vi "RT - Initialize Control Mode.vi"(8 "error in":errorcluster) -> (0 "error out":errorcluster)   [LabVIEW 2014]
uses:
  Controls/DLT State.ctl
  Controls/IT State.ctl
  Controls/OT State.ctl
  Controls/TWT State.ctl
  Controls/Clean State.ctl
  Controls/DL State.ctl
  Controls/Clamp State.ctl
  Controls/BR State.ctl
  Controls/ConfigCalibration.ctl
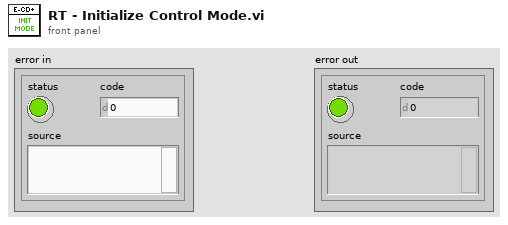
[diagram p1: front panel]
types:
  T1 = typedef "ConfigCalibration.ctl" = enum16{"CAL STOP", "TWTT OP (IN)", "TWTT PDP (IN)", "DLT OP (IN)", "DLT PDP 01 (IN)", "DLT PDP 02 (IN)", "BR OP (IN)", "BR TWT ALIGN (IN)", "BR DL ALIGN (IN)"}
  T2 = typedef "Clean State.ctl" = enum16{"CLEAN STOP", "CLEAN CAMERA", "CLEAN THREADS", "CLEAN THREADS MANUAL", "SV-12 H2O PILOT TRUE", "SV-12 H2O PILOT FALSE", "SV-13 CLEAN AIR TRUE", "SV-13 CLEAN AIR FALSE", "SV-15 CLEAN H2O TRUE", "SV-15 CLEAN H2O FALSE"}
  T3 = typedef "DLT State.ctl" = enum16{"DLT STOP", "DLT DRIVE FWD PDP", "DLT DRIVE FWD", "DLT DRIVE BWD", "DLT DRIVE BWD PDP CLEAN", "DLT DRIVE BWD PDP", "DLT HOLD BACK", "SV-7 DLT FWD TRUE", "SV-7 DLT FWD FALSE", "SV-8 DLT BWD TRUE", "SV-8 DLT BWD FALSE", "DLT RESET"}
  T4 = typedef "DL State.ctl" = enum16{"DL STOP", "DL ROTATE CW", "DL ROTATE CCW", "SV-3 DL CW TRUE", "SV-3 DL CW FALSE", "SV-3 DL CCW TRUE", "SV-3 DL CCW FALSE"}
  T5 = typedef "TWT State.ctl" = enum16{"TWTT STOP", "TWTT DRIVE FWD PDP", "TWTT DRIVE BWD PDP", "TWTT BWD 0.256 IN", "TWTT FWD 0.256 IN", "TWT FWD BEFORE SCREW", "SV-5 TWTT FWD TRUE", "SV-5 TWTT FWD FALSE", "SV-6 TWTT BWD TRUE", "SV-6 TWTT BWD FALSE", "TWTT RESET"}
  T6 = typedef "OT State.ctl" = enum16{"OT STOP", "OT ROTATE CW ENG", "OT ROTATE CCW 2.5 REV", "OT ROTATE CW 2.5 REV", "OT CW TIGHTEN PLUG", "SV-2 OT CW TRUE", "SV-2 OT CW FALSE", "SV-2 OT CCW TRUE", "SV-2 OT CCW FALSE"}
  T7 = typedef "IT State.ctl" = enum16{"IT STOP", "IT ROTATE CCW ENG", "IT ROTATE CCW QF1R", "IT CCW ENG & QF1R", "IT ROTATE CCW 2.5 REV", "IT ROTATE CW 2.5 REV", "IT CW TIGHTEN VALVE", "IT CCW PULSE", "SV-1 IT CW TRUE", "SV-1 IT CW FALSE", "SV-1 IT CCW TRUE", "SV-1 IT CCW FALSE"}
  T8 = typedef "BR State.ctl" = enum16{"BR STOP", "BR DRIVE LEFT PDP", "BR LEFT ALIGN TWT", "BR DRIVE RIGHT PDP", "BR RIGHT TO INIT", "BR RIGHT FOR DL", "SV-4 BR RIGHT TRUE", "SV-4 BR RIGHT FALSE", "SV-4 BR LEFT TRUE", "SV-4 BR LEFT FALSE", "BR RESET"}
  T9 = typedef "Clamp State.ctl" = enum16{"CLAMP STOP", "CLAMP CLOSE", "CLAMP OPEN"}
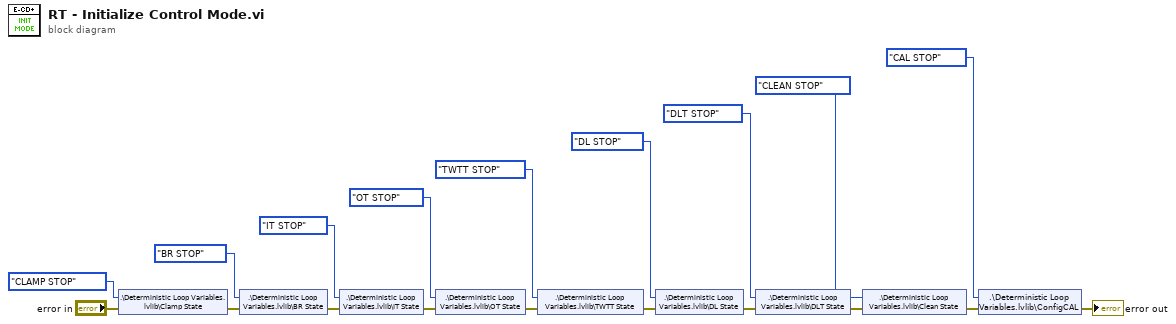
[diagram p0: block diagram]
diagram:
  n1 = shared-variable ".\\Deterministic Loop Variables.lvlib\\Clamp State"(Clamp_State."CLAMP STOP" ("Clamp State"), error in="error in") -> (error out=w13:errorcluster)
  n2 = shared-variable ".\\Deterministic Loop Variables.lvlib\\BR State"(BR_State."BR STOP" ("BR State"), error in=w13) -> (error out=w19:errorcluster)
  n3 = shared-variable ".\\Deterministic Loop Variables.lvlib\\IT State"(IT_State."IT STOP" ("IT State"), error in=w19) -> (error out=w18:errorcluster)
  n4 = shared-variable ".\\Deterministic Loop Variables.lvlib\\OT State"(OT_State."OT STOP" ("OT State"), error in=w18) -> (error out=w17:errorcluster)
  n5 = shared-variable ".\\Deterministic Loop Variables.lvlib\\TWTT State"(TWT_State."TWTT STOP" ("TWTT State"), error in=w17) -> (error out=w16:errorcluster)
  n6 = shared-variable ".\\Deterministic Loop Variables.lvlib\\DL State"(DL_State."DL STOP" ("DL State"), error in=w16) -> (error out=w15:errorcluster)
  n7 = shared-variable ".\\Deterministic Loop Variables.lvlib\\DLT State"(DLT_State."DLT STOP" ("DLT State"), error in=w15) -> (error out=w14:errorcluster)
  n8 = shared-variable ".\\Deterministic Loop Variables.lvlib\\Clean State"(Clean_State."CLEAN STOP" ("Clean State"), error in=w14) -> (error out=w3:errorcluster)
  n9 = shared-variable ".\\Deterministic Loop Variables.lvlib\\ConfigCAL"(ConfigCalibration."CAL STOP" ("ConfigCAL"), error in=w3) -> (error out=→"error out":errorcluster)
